vi "Playback Frame.vi"(8 "error in (no error)":errorcluster, 10 "Recording Settings":T1={"Folder to Save Recording"=path "", "Recording Name"="", "Video FPS"=1.0, "Codec"=0, "Operator"=0, "Tracker FPS"=1.0} {"Tracker FPS" min=0.0 max=100.0; "Operator" items=["Novice", "Expert"]; "Codec" items=["Cinepak Codec by Radius", "Intel IYUV codec", "Microsoft Video 1", "FF Video Codec 1 (FFV1) (NI Vision)", "Motion JPEG (NI Vision)", "Y800 Uncompressed Grey Scale (NI Vision)", "YUV 4:2:0 Planar (NI Vision)"]; "Video FPS" min=0.0 max=100.0}, 11 "Frame Grabber Data in":T3) -> (0 "error out":errorcluster, 1 "Presentation":string, 2 "Image":T2, 3 "Frame Grabber Data out":T3, 4 "Time elapsed (s)":dbl)   [LabVIEW 2017]
uses:
  Controls/Frame Grabber Data.ctl
  <vilib>/userdefined/High Color/IMAQdx.ctl
  <vilib>/vision/Image Controls.llb/IMAQ Image.ctl
  <vilib>/vision/Avi.llb/IMAQ AVI2 Refnum.ctl
  Controls/Rigid Body Info.ctl
  Controls/Position.ctl
  Controls/Orientation.ctl
  Controls/Recording Settings.ctl
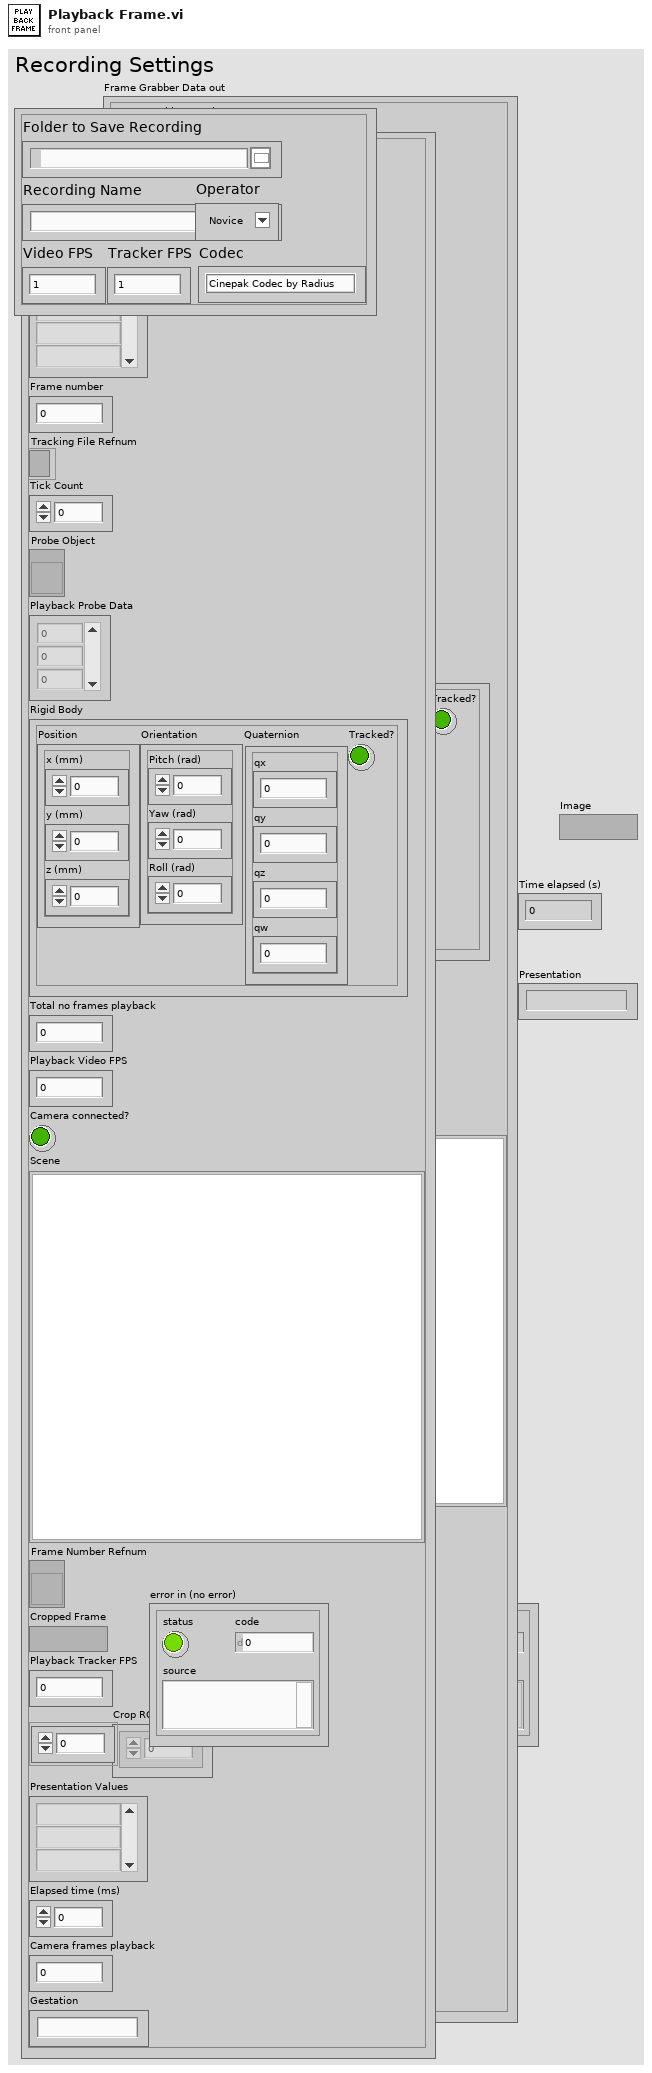
[diagram p1: front panel]
types:
  T1 = typedef "Recording Settings.ctl" = cluster{"Folder to Save Recording":path, "Recording Name":string, "Video FPS":dbl, "Codec":u16, "Operator":u16, "Tracker FPS":dbl}
  T2 = typedef "IMAQ Image.ctl" = refnum<image>
  T3 = typedef "Frame Grabber Data.ctl" = cluster{"Camera Session":T4, "Frame":T2, "AVI Refnum":T5, "Codecs":string[], "Frame number":u32, "Tracking File Refnum":refnum<file>, "Tick Count":u32, "Probe Object":refnum<vi>, "Playback Probe Data":dbl[][], "Rigid Body":T6, "Total no frames playback":u32, "Playback Video FPS":u32, "Camera connected?":bool, "Scene":refnum<vi>, "Frame Number Refnum":refnum<vi>, "Cropped Frame":T2, "Playback Tracker FPS":u32, "Crop ROI":i32[], "Presentation Values":string[], "Elapsed time (ms)":u32, "Camera frames playback":u32, "Gestation":string}
  T4 = typedef "IMAQdx.ctl" = refnum<k21>
  T5 = typedef "IMAQ AVI2 Refnum.ctl" = refnum<k20>
  T6 = typedef "Rigid Body Info.ctl" = cluster{"Position":T7, "Orientation":T8, "Quaternion":cluster{"qx":sgl, "qy":sgl, "qz":sgl, "qw":sgl}, "Tracked?":bool}
  T7 = typedef "Position.ctl" = cluster{"x (mm)":sgl, "y (mm)":sgl, "z (mm)":sgl}
  T8 = typedef "Orientation.ctl" = cluster{"Pitch (rad)":sgl, "Yaw (rad)":sgl, "Roll (rad)":sgl}
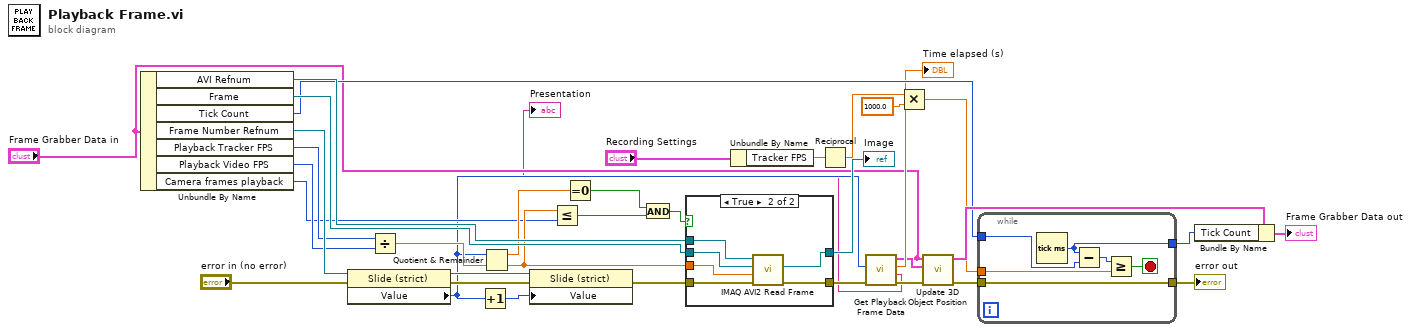
[diagram p0: block diagram]
diagram:
  n1 = Unbundle By Name("Frame Grabber Data in") -> ("AVI Refnum"=w34:T5, "Frame"=w35:T2, "Tick Count"=w25:u32, "Frame Number Refnum"=w23:refnum<vi>, "Playback Tracker FPS"=w16:u32, "Playback Video FPS"=w15:u32, "Camera frames playback"=w12:u32)
  n2 = property class="Slide (strict)"(reference=w23, error in="error in (no error)") -> (reference out=w21:refnum<vi>, error out=w9:errorcluster, "Value"=w6:u32)
  n3 = Divide(x=w16, y=w15) -> (x/y=w14:dbl)
  n4 = Increment(x=w6) -> (x+1=w22:u32)
  n5 = Quotient & Remainder(x=w6, y=w14) -> (x-y*floor(x/y)=w18:dbl, floor(x/y)=w13:dbl)
  n6 = property class="Slide (strict)"(reference=w21, error in=w9, "Value"=w22) -> (error out=w8:errorcluster)  [unwired: 1 out]
  n7 = Less Or Equal?(x=w13, y=w12) -> (x <= y?=w10:bool)
  n8 = Equal To 0?(x=w18) -> (x = 0?=w17:bool)
  n9 = And(x=w17, y=w10) -> (x .and. y?=w11:bool)
  n10 = case shown="True" w11 {
    tunnel: [w37 w44] -> w36
    tunnel: w35 -> [w37 w43]
    tunnel: w34 -> [_ w42]
    tunnel: [w38 w41] -> w5
    tunnel: w8 -> [w38 w40]
    tunnel: w13 -> [_ w39]
    frame False {
    }
    frame True {
      n11 = call "IMAQ AVI2 Read Frame"("error in (no error)"=w40, "Frame Number"=w39, "Image"=w43, "AVI Refnum"=w42) -> ("error out"=w41:errorcluster, "Image Out"=w44:T2)  [unwired: 5 in, 1 out]
    }
  }
  "Image" <- w36
  n12 = Unbundle By Name("Recording Settings") -> ("Tracker FPS"=w19:dbl)
  n13 = Reciprocal(x=w19) -> (1/x=w28:dbl)
  n14 = call "Get Playback Frame Data.vi"("Error In"=w5, "Frame number"=w6, "Frame Grabber Data"="Frame Grabber Data in") -> ("Error Out"=w4:errorcluster, "Presentation"=→"Presentation":string, "Time elapsed (s)"=→"Time elapsed (s)":dbl, "New Rigid Body Position"=w3:T6)  [unwired: 4 in, 1 out]
  n15 = Multiply(x=w28, y=1000.0) -> (x*y=w26:dbl)
  n16 = call "Update 3D Object Position.vi"("error in (no error)"=w4, "New Rigid Body Position"=w3, "Frame Grabber Data in"="Frame Grabber Data in") -> ("error out"=w31:errorcluster, "Frame Grabber Data out"=w32:T3)  [unwired: 7 in]
  n17 = while {
    tunnel: [w50] -> w29
    tunnel: w26 -> [w47]
    tunnel: w25 -> [w46]
    tunnel: w31 -> [w45]
    tunnel: [w45] -> w30
    stop <- w49 stop-if-true
    n18 = Tick Count (ms)() -> (millisecond timer value=w50:u32)
    n19 = Subtract(x=w50, y=w46) -> (x-y=w48:u32)
    n20 = Greater Or Equal?(x=w48, y=w47) -> (x >= y?=w49:bool)
  }
  "error out" <- w30
  n21 = Bundle By Name(cluster=w32, "Tick Count"=w29) -> (→"Frame Grabber Data out":T3)
